vi "Start Driver Server.vi"(8 "error in (no error)":errorcluster) -> (0 "error out":errorcluster)   [LabVIEW 2010]
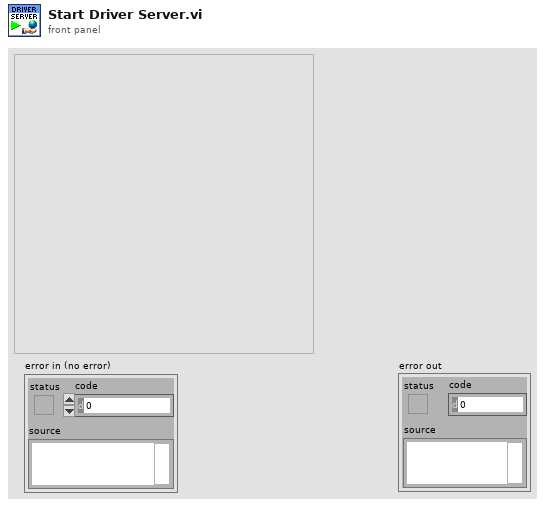
[diagram p1: front panel]
types:
  T1 = typedef "Path InitDynamicVIsPaths__FS.ctl" = cluster{"F4 Operation":path, "F4 Alarms":path, "F4 Inputs":path, "F4 Outputs":path, "F4 PID Sets":path, "F4 Cascade":path, "F4 Current Step":path, "Profile SubPanel":path, "Profile Editor":path, "MainVI":path, "Profile Control":path, "Synergy Control":path, "Driver Server":path}
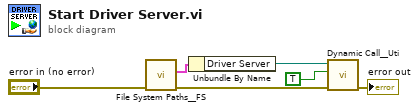
[diagram p0: block diagram]
diagram:
  n1 = call "File System Paths__FS.vi"("error in (no error)"="error in (no error)") -> ("error out"=w6:errorcluster, "DynamicVIs"=w3:T1)  [unwired: 8 in, 1 out]
  n2 = Unbundle By Name(w3) -> ("Driver Server"=w4:path)
  n3 = call "Dynamic Call__Uti.vi"("error in (no error)"=w6, "open front panel? (T)"=TRUE, "vi path"=w4) -> ("error out"=→"error out":errorcluster)  [unwired: 8 in]
